vi "Roll Die.vi"() -> (3 "Number":i32)   [LabVIEW 2015]
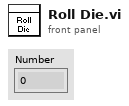
[diagram p1: front panel]
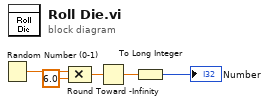
[diagram p0: block diagram]
diagram:
  n1 = Random Number (0-1)() -> (number: 0 to 1=w5:dbl)
  n2 = Compound Arithmetic op=MULTIPLY(w5, 6.0 ("value")) -> (w3:dbl)
  n3 = Round Toward -Infinity(1:w3) -> (0:w2:dbl)
  n4 = To Long Integer(number=w2) -> (32bit integer=→"Number":i32)
